vi "checkIfPositionIsInField.vi"(8 "error in (no error)":errorcluster, 9 "Position":dbl[](array[numeric]), 10 "FieldRef":refnum<class "Field.lvclass">, 11 "Utilities in":refnum<class "Utilities.lvclass">) -> (0 "error out":errorcluster, 2 "Position Is In Field?":bool, 3 "Utilities out":refnum<class "Utilities.lvclass">, 4 "y Is in Field?":bool, 6 "x Is in Field?":bool)   [LabVIEW 2020, in "Utilities.lvclass"]
uses:
  Utilities.lvclass
  Field_class/Field.lvclass
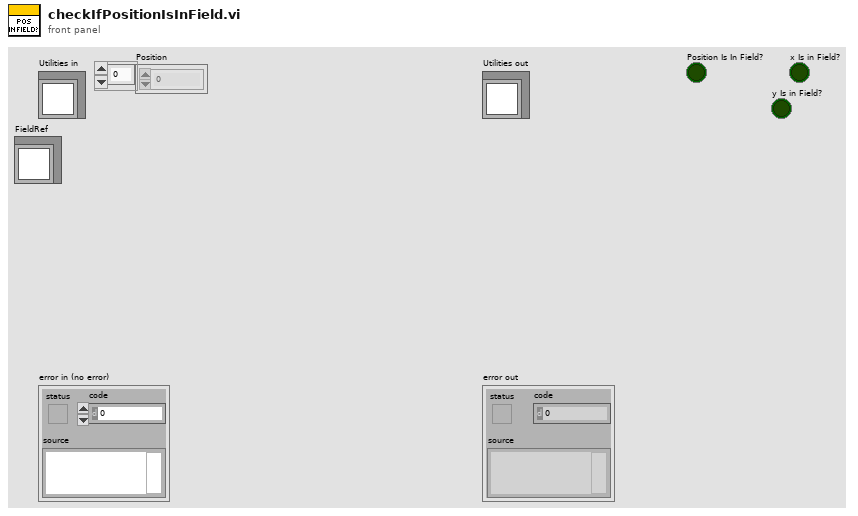
[diagram p1: front panel]
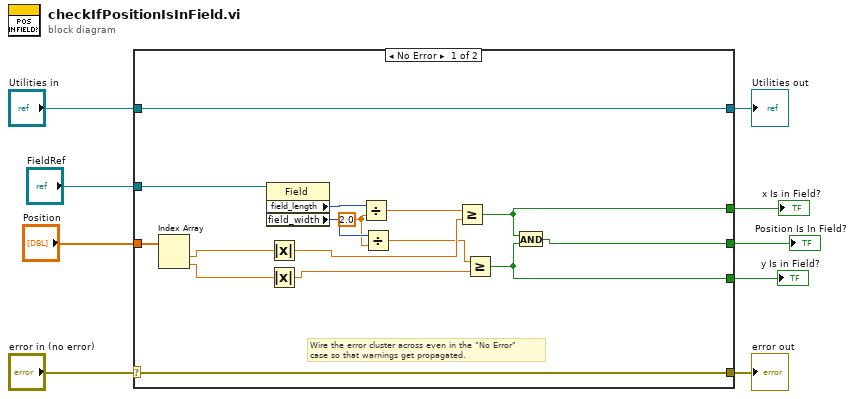
[diagram p0: block diagram]
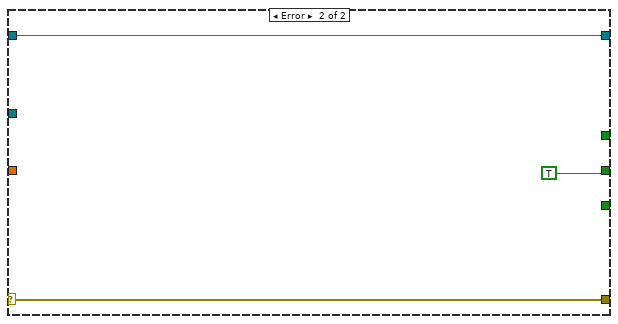
[diagram p2: hidden frame]
diagram:
  n1 = case shown="No Error" "error in (no error)" {
    selector: "error in (no error)" -> [w24 w28]
    tunnel: [w24 w28] -> w8
    tunnel: [w25 w27] -> w6
    tunnel: "Utilities in" -> [w25 w27]
    tunnel: "Position" -> [w23 _]
    tunnel: [w13 TRUE] -> w4
    tunnel: [w12 _] -> w3
    tunnel: [w11 _] -> w2
    tunnel: "FieldRef" -> [w10 _]
    frame No Error {
      w18 = 2.0
      # "Wire the error cluster across even in the \"No Error\"\ncase so that warnings get propagated."
      n2 = Index Array(array=w23) -> (element #1=w22:dbl, element #2=w21:dbl)  [unwired: 2 in]
      n3 = property class="Field"(reference=w10) -> ("field_length"=w20:i32, "field_width"=w19:i32)  [unwired: 1 in, 2 out]
      n4 = Absolute Value(x=w22) -> (abs(x)=w16:dbl)
      n5 = Absolute Value(x=w21) -> (abs(x)=w14:dbl)
      n6 = Divide(x=w20, y=w18) -> (x/y=w17:dbl)
      n7 = Divide(x=w19, y=w18) -> (x/y=w15:dbl)
      n8 = Greater Or Equal?(x=w17, y=w16) -> (x >= y?=w12:bool)
      n9 = Greater Or Equal?(x=w15, y=w14) -> (x >= y?=w11:bool)
      n10 = And(x=w12, y=w11) -> (x .and. y?=w13:bool)
    }
    frame Error {
    }
  }
  "error out" <- w8
  "Utilities out" <- w6
  "Position Is In Field?" <- w4
  "x Is in Field?" <- w3
  "y Is in Field?" <- w2
